vi "E816_Simple_Test.vi"() -> ()   [LabVIEW 2011]
doc: "This simple test VI is a stand-alone sample application. \nSpecify first: \n¢ System no. (= 1 in a one-system configuration),\n¢ Timeout value (im milliseconds)\n¢ Portnumber\n¢ Baudrate. If you don't know the baudrate settings of the connected E-816, leave Try different baudrates? TRUE. The VI will then try to find the correct baudrate automatically by calling \"Find baudrate.vi\".\nThen start the VI. The VI will open a connection to the E-816 and query the controller for the available axis IDs, position values of these axes, and the master E-816 identification string. The diagram shows how to combine the driver and support VIs for these tasks."
panel:
  in  "RS-232 Portnumber":i32(ring) items=["COM1", "COM2", "COM3", "COM4", "COM5", "COM6", "COM7", "COM8", "COM9", "COM10", "COM11", "COM12", "COM13", "COM14", "COM15", "COM16", "COM17", "COM18", "COM19", "COM20", "COM21", "COM22", "COM23", "COM24", "COM25", "COM26", "COM27", "COM28", "COM29", "COM30"]
  in  "error in":errorcluster
  in  "System no.":i32=1 min=1 max=4 step=1
  in  "Wait":string="Please wait.\nChecking for correct baudrate."
  in  "Try different baudrates?":bool=TRUE
  in  "RS-232 Baudrate":u16(ring)=4 items=["9600", "14400", "19200", "38400", "57600", "115200"]
  in  "Timeout":i32=5000
  out "error out":errorcluster
  out "Position":dbl[](array[numeric]) format="%.6f"
  out "Conn. Axes":string[](array[string])
  out "Identification":string="\n"
  # "Simple E-816 communication test program"
  # "Select Portnumber, Baudrate and timeout value first, then start the VI. If you\ndon't know the correct Baudrate, leave \"Try different baudrates?\" TRUE. \nThen start the VI. The VI will open the chosen port, query for connected axes (SAI?), position (POS?), and\nmaster E-816 Identification (*IDN?). See VI and control/ indicator information for details."
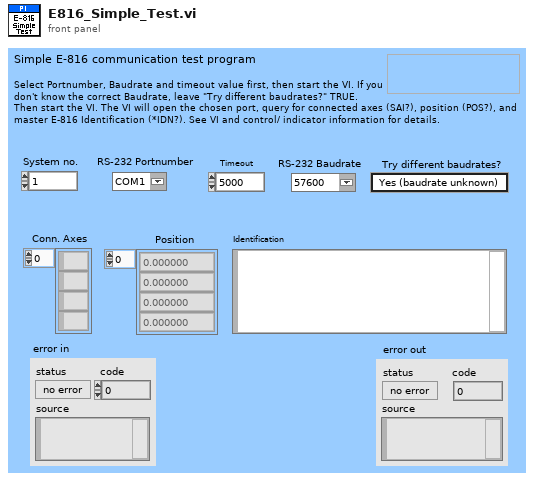
[diagram p1: front panel]
types:
  T1 = enum16{"DCO", "DCO?", "MOV", "MOV?", "MVR", "ONT?", "OVF?", "POS?", "RST", "SVA", "SVA?", "SVO", "SVO?", "SVR", "VOL?"}
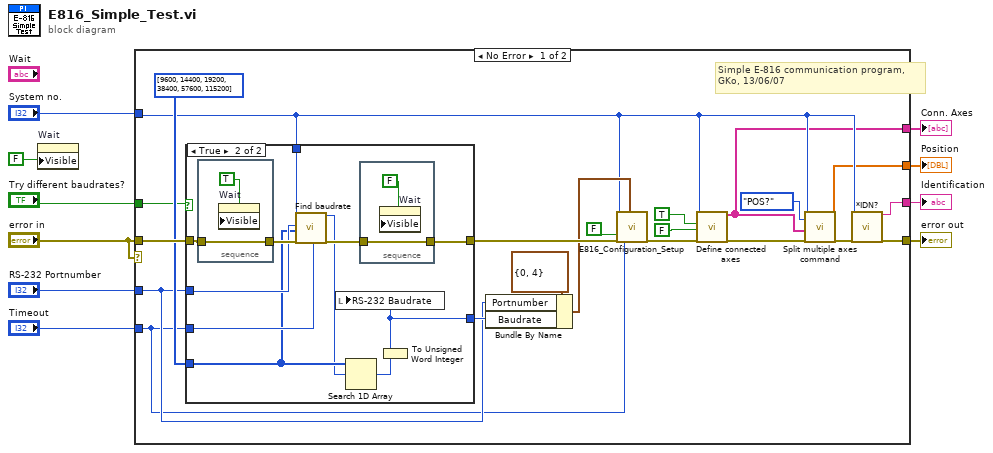
[diagram p0: block diagram]
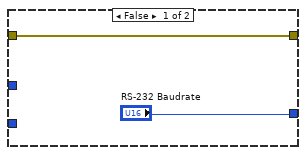
[diagram p2: hidden frame]
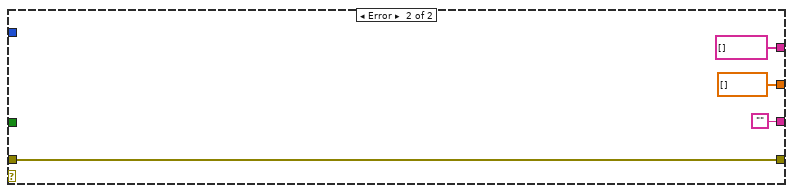
[diagram p3: hidden frame]
diagram:
  n1 = property on="Wait" class="Str"("Visible"=FALSE ("Write Attribute")) -> ()  [unwired: 2 in, 2 out]
  n2 = case shown="No Error" "error in" {
    tunnel: [w28 w52] -> w10
    tunnel: "error in" -> [w27 w52]
    tunnel: "System no." -> [w19 _]
    tunnel: "Try different baudrates?" -> [w18 _]
    tunnel: "RS-232 Portnumber" -> [w17 _]
    tunnel: "Timeout" -> [w16 _]
    tunnel: [w15 "" ("Identification")] -> w3
    tunnel: [w14 dbl[] [] ("Num. values out")] -> w2
    tunnel: [w13 string[] [] ("Conn. Axes out")] -> w1
    frame No Error {
      # "Simple E-816 communication program,\nGKo, 13/06/07"
      n3 = case shown="True" w18 {
        tunnel: ["RS-232 Baudrate" w34] -> w21
        tunnel: [w33 w44] -> w25
        tunnel: w27 -> [w33 w43]
        tunnel: w16 -> [_ w40]
        tunnel: w17 -> [_ w39]
        tunnel: w19 -> [_ w38]
        tunnel: u32[] [9600, 14400, 19200, 38400, 57600, 115200] ("Valid Baudrates") -> [_ w36]
        frame False {
        }
        frame True {
          n4 = stacked-sequence {
            tunnel: w43 -> [w46]
            tunnel: [w46] -> w41
            frame #0 {
              n5 = property on="Wait" class="Str"("Visible"=TRUE ("Write Attribute")) -> ()  [unwired: 2 in, 2 out]
            }
          }
          n6 = call "Find baudrate.vi"("System no."=w38, "RS-232 Portnumber"=w39, "Valid Baudrates"=w36, "error in"=w41, "Timeout"=w40) -> ("Baudrate out"=w35:u32, "error out"=w42:errorcluster)  [unwired: 12 in, 1 out]
          n7 = Search 1D Array(1D array=w36, element=w35) -> (index of element=w37:i32)  [unwired: 1 in]
          n8 = stacked-sequence {
            tunnel: w42 -> [w47]
            tunnel: [w47] -> w44
            frame #0 {
              n9 = property on="Wait" class="Str"("Visible"=FALSE ("Write Attribute")) -> ()  [unwired: 2 in, 2 out]
            }
          }
          n10 = To Unsigned Word Integer(number=w37) -> (unsigned 16bit integer=w34:u16)
          n11 = local write "RS-232 Baudrate"(w34) -> ()
        }
      }
      n12 = Bundle By Name(cluster=cluster{"Portnumber":i32, "Baudrate":u16} {"Portnumber"=0, "Baudrate"=4} ("RS232 settings"), "Portnumber"=w17, "Baudrate"=w21) -> (w23:cluster{"Portnumber":i32, "Baudrate":u16})
      n13 = call "E816_Configuration_Setup.vi"("System no."=w19, "Change servo \nstatus to ON?"=FALSE ("Change servo \nstatus to ON?"), "error in"=w25, "Timeout"=w16, "RS232 settings"=w23) -> ("error out"=w26:errorcluster)  [unwired: 11 in, 3 out]
      n14 = call "Define connected axes.vi"("System no."=w19, "Read from\ncontroller?"=TRUE ("Read from\nController"), "Invert\norder?"=FALSE ("Invert\nOrder"), "error in"=w26) -> ("Conn. Axes out"=w13:string[], "error out"=w29:errorcluster)  [unwired: 14 in]
      n15 = call "Split multiple axes command.vi"("System no."=w19, "Command"=T1."POS?", "Axes to command"=w13, "error in"=w29) -> ("Num. values out"=w14:dbl[], "error out"=w24:errorcluster)  [unwired: 13 in, 1 out]
      n16 = call "*IDN?.vi"("System no."=w19, "error in"=w24) -> ("Identification"=w15:string, "error out"=w28:errorcluster)  [unwired: 16 in]
    }
    frame Error {
    }
  }
  "error out" <- w10
  "Identification" <- w3
  "Position" <- w2
  "Conn. Axes" <- w1
